vi "Determine Code Transition Values.vi"(7 "Transition":dbl, 8 "Intercept":dbl, 9 "Slope":dbl, 10 "End":dbl, 11 "Start":dbl) -> (1 "Calculated transition":dbl, 2 "Actual end":dbl, 3 "Actual start":dbl)   [LabVIEW 2021, in "adc_fullScaleError.lvlib"]
uses:
  adc_fullScaleError.lvlib
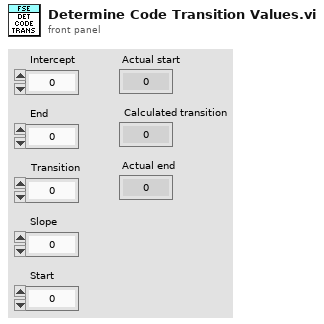
[diagram p1: front panel]
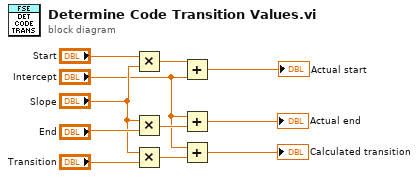
[diagram p0: block diagram]
diagram:
  n1 = Multiply(x="Start", y="Slope") -> (x*y=w10:dbl)
  n2 = Multiply(x="Slope", y="End") -> (x*y=w7:dbl)
  n3 = Multiply(x="Slope", y="Transition") -> (x*y=w3:dbl)
  n4 = Add(x=w10, y="Intercept") -> (x+y=→"Actual start":dbl)
  n5 = Add(x="Intercept", y=w7) -> (x+y=→"Actual end":dbl)
  n6 = Add(x="Intercept", y=w3) -> (x+y=→"Calculated transition":dbl)
